vi "Update Cycle Count.vi"(8 "error in (no error)":errorcluster, 11 "Worker in":refnum<class "Worker Actor.lvclass">) -> (0 "error out":errorcluster, 2 "Cycle count out":i32, 3 "Worker out":refnum<class "Worker Actor.lvclass">)   [LabVIEW 2021, in "Worker Actor.lvclass"]
uses:
  Worker Actor.lvclass
  Worker Actor.lvclass/Worker Actor.ctl
  Read Cycle count.vi
  Write Cycle count.vi
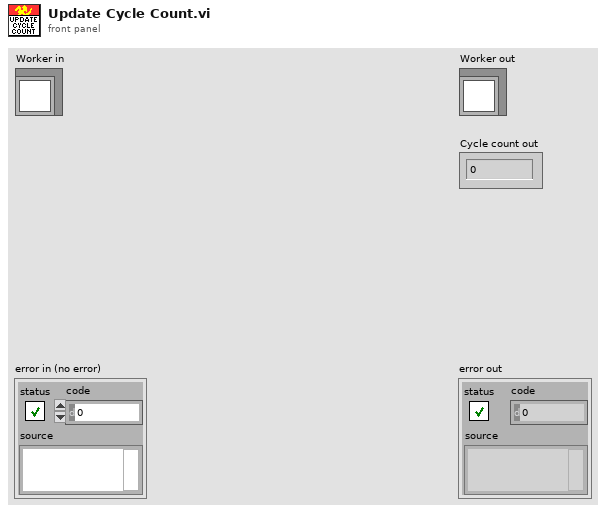
[diagram p1: front panel]
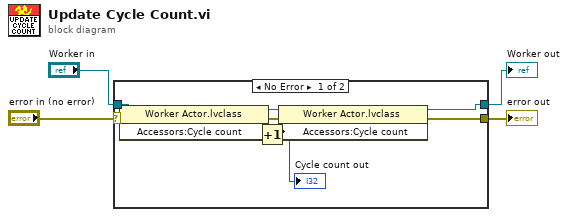
[diagram p0: block diagram]
diagram:
  n1 = case shown="No Error" "error in (no error)" {
    selector: "error in (no error)" -> [w12 w14]
    tunnel: [w9 w14] -> w3
    tunnel: [w7 w13] -> w1
    tunnel: "Worker in" -> [w10 w13]
    frame No Error {
      n2 = property class="Worker Actor.lvclass"(reference=w10, error in=w12) -> (reference out=w8:refnum<class "Worker Actor.lvclass">, error out=w11:errorcluster, "Accessors:Cycle count"=w6:i32)
      n3 = Increment(x=w6) -> (x+1=w5:i32)
      "Cycle count out" <- w5
      n4 = property class="Worker Actor.lvclass"(reference=w8, error in=w11, "Accessors:Cycle count"=w5) -> (reference out=w7:refnum<class "Worker Actor.lvclass">, error out=w9:errorcluster)
    }
    frame Error {
    }
  }
  "error out" <- w3
  "Worker out" <- w1
